vi "Send ADC.vi"(8 "error in (no error)":errorcluster, 9 "Channel":enum16{"2", "1"}(ring), 10 "VISA resource name":refnum<visa-resource-name>, 11 "Simulated Device in":refnum<class "Simulated Device.lvclass">) -> (0 "error out":errorcluster, 1 "Response":i32, 2 "VISA resource name 2":refnum<visa-resource-name>, 3 "Simulated Device out":refnum<class "Simulated Device.lvclass">)   [LabVIEW 2020, in "Simulated Device.lvclass"]
uses:
  Simulated Device.lvclass
  Abstract/Serial Device/Serial Device.lvclass
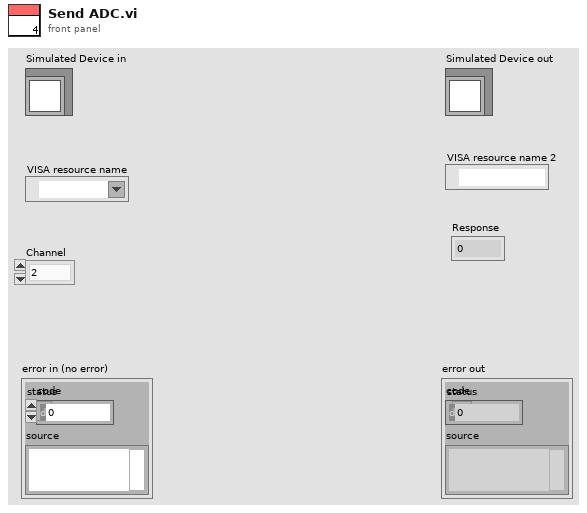
[diagram p1: front panel]
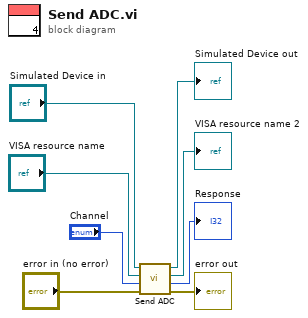
[diagram p0: block diagram]
diagram:
  n1 = call-parent "Send ADC.vi"("error in (no error)"="error in (no error)", "Channel"="Channel", "VISA resource name"="VISA resource name", "Serial Device in"="Simulated Device in") -> ("error out"=→"error out":errorcluster, "Response"=→"Response":i32, "VISA resource name 2"=→"VISA resource name 2":refnum<visa-resource-name>, "Serial Device out"=→"Simulated Device out":refnum<class "Simulated Device.lvclass">)  [unwired: 4 in]
